vi "TagCreatePixelArrayV1Tags.vi"(5 "Layout":string, 7 "Codes":i64[](array[numeric]), 8 "error in (no error)":errorcluster, 11 "ID":i32) -> (0 "error out":errorcluster, 3 "Pixels":u8[][](array[numeric]))   [LabVIEW 2020, in "g_ar_toolkit.feature_detection.lvlib"]
uses:
  g_ar_toolkit.feature_detection.lvlib
  TagPixelType.ctl
  <vilib>/Utility/error.llb/Error Cluster From Error Code.vi
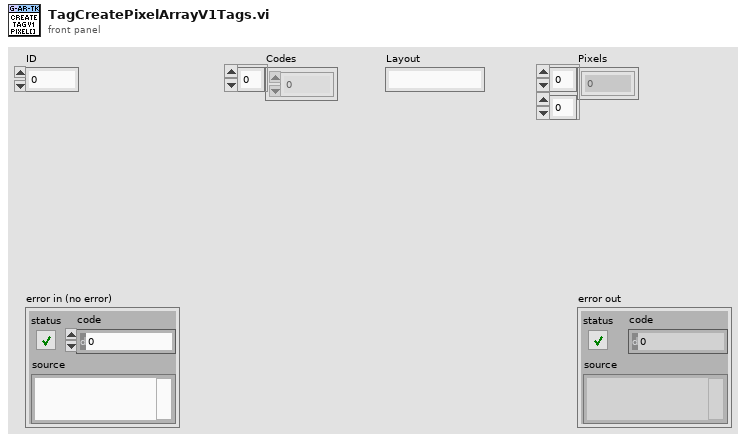
[diagram p1: front panel]
types:
  T1 = typedef "g_ar_toolkit.feature_detection.lvlib/TagPixelType.ctl" = enum8{"Black", "White", "Transparent"}
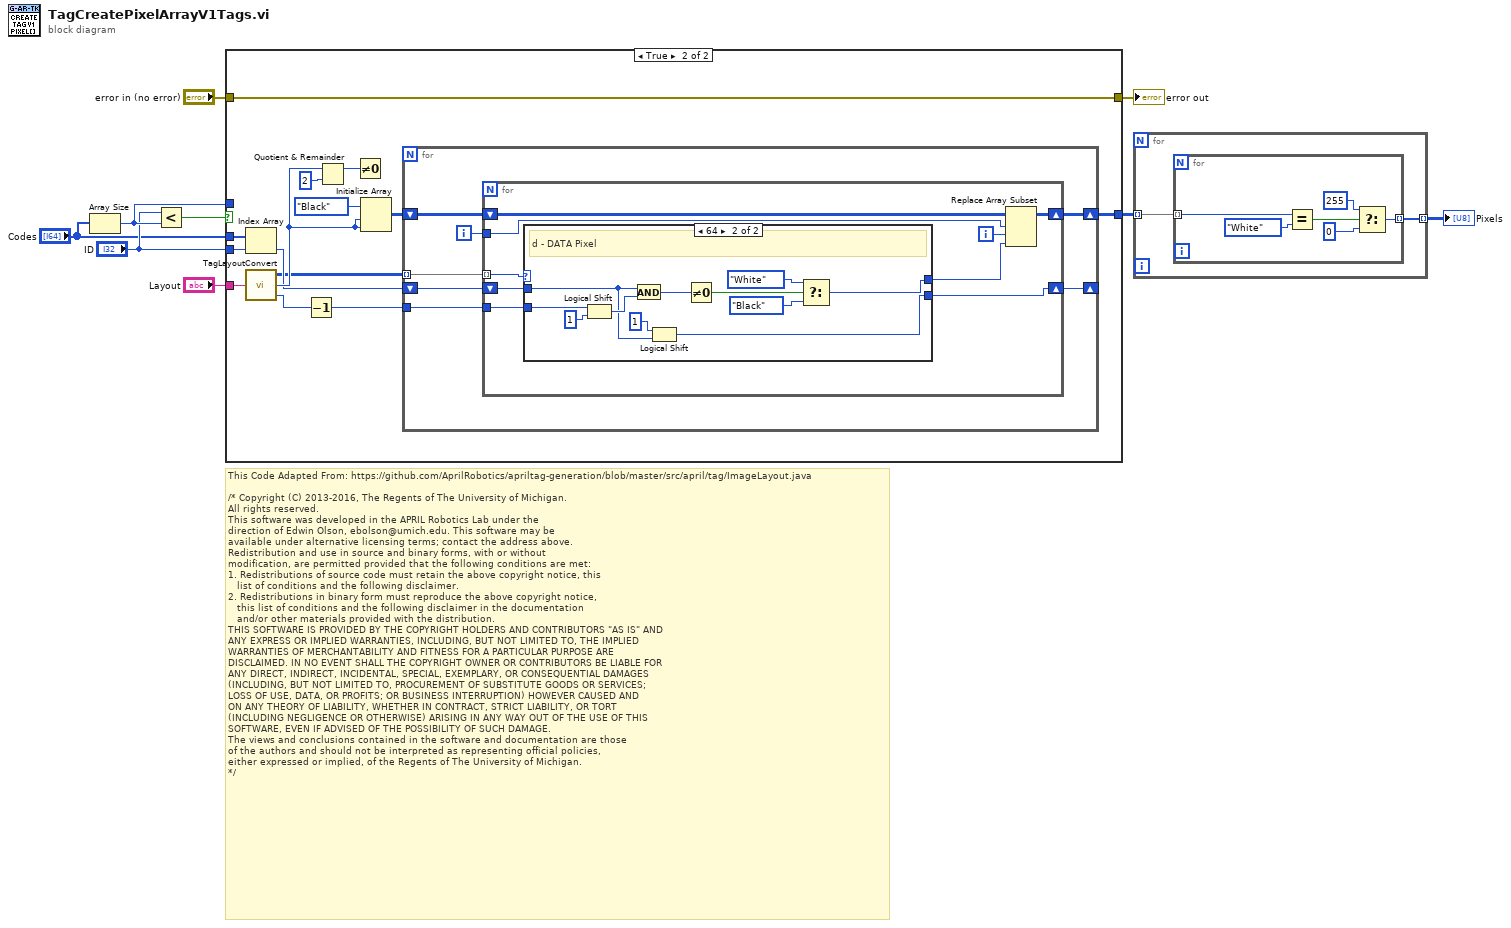
[diagram p0: block diagram]
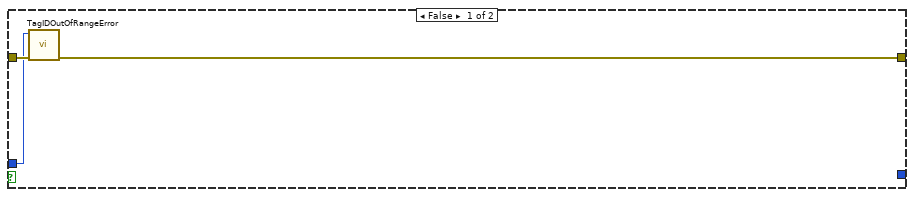
[diagram p2: hidden frame]
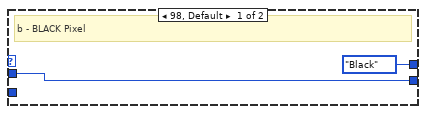
[diagram p3: hidden frame]
diagram:
  # "This Code Adapted From: https://github.com/AprilRobotics/apriltag-generation/blob/master/src/april/tag/ImageLayout.java\n\n/* Copyright (C) 2013-2016, The Regents of The University of Michigan.\nAll rights reserved.\nThis software was developed in the APRIL Robotics Lab under the\ndirection of Edwin Olson, ebolson@umich.edu. This software may be\navailable under alternative licensing terms; contact the address above.\nRedistribution and use in source and binary forms, with or without\nmodification, are permitted provided that the following conditions are met:\n1. Redistributions of source code must retain the above copyright notice, this\n   list of conditions and the following disclaimer.\n2. Redistributions in binary form must reproduce the above copyright notice,\n   this list of conditions and the following disclaimer in the documentation\n   and/or other materials provided with the distribution.\nTHIS SOFTWARE IS PROVIDED BY THE COPYRIGHT HOLDERS AND CONTRIBUTORS \"AS IS\" AND\nANY EXPRESS OR IMPLIED WARRANTIES, INCLUDING, BUT NOT LIMITED TO, THE IMPLIED\nWARRANTIES OF MERCHANTABILITY AND FITNESS FOR A PARTICULAR PURPOSE ARE\nDISCLAIMED. IN NO EVENT SHALL THE COPYRIGHT OWNER OR CONTRIBUTORS BE LIABLE FOR\nANY DIRECT, INDIRECT, INCIDENTAL, SPECIAL, EXEMPLARY, OR CONSEQUENTIAL DAMAGES\n(INCLUDING, BUT NOT LIMITED TO, PROCUREMENT OF SUBSTITUTE GOODS OR SERVICES;\nLOSS OF USE, DATA, OR PROFITS; OR BUSINESS INTERRUPTION) HOWEVER CAUSED AND\nON ANY THEORY OF LIABILITY, WHETHER IN CONTRACT, STRICT LIABILITY, OR TORT\n(INCLUDING NEGLIGENCE OR OTHERWISE) ARISING IN ANY WAY OUT OF THE USE OF THIS\nSOFTWARE, EVEN IF ADVISED OF THE POSSIBILITY OF SUCH DAMAGE.\nThe views and conclusions contained in the software and documentation are those\nof the authors and should not be interpreted as representing official policies,\neither expressed or implied, of the Regents of The University of Michigan.\n*/"
  n1 = Array Size(array="Codes") -> (size(s)=w8:i32)
  n2 = Less?(x="ID", y=w8) -> (x < y?=w5:bool)
  n3 = case shown="True" w5 {
    tunnel: "Codes" -> [_ w26]
    tunnel: "ID" -> [_ w25]
    tunnel: "error in (no error)" -> [w12 w19]
    tunnel: [w11 w19] -> w7
    tunnel: w8 -> [w10 _]
    tunnel: "Layout" -> [_ w21]
    tunnel: [_ w13] -> w2
    frame False {
      n4 = call "TagIDOutOfRangeError.vi"("error in (no error)"=w12, "Tag Family Size"=w10) -> ("error out"=w11:errorcluster)  [unwired: 9 in]
    }
    frame True {
      n5 = Index Array(array=w26, index=w25) -> (element=w18:i64)
      n6 = call "TagLayoutConvert.vi"("Layout"=w21) -> ("Pixel Map"=w17:u8[][], "Size"=w20:i32, "Number Of Bits"=w15:i32)
      n7 = Decrement(x=w15) -> (x-1=w14:i32)
      n8 = Quotient & Remainder(x=w20, y=2) -> (x-y*floor(x/y)=w23:i32)  [unwired: 1 out]
      n9 = Not Equal To 0?(x=w23) -> ()  [unwired: 1 out]
      n10 = Initialize Array(TagPixelType."Black", w20, w20) -> (w16:T1[][])
      n11 = for {
        shift-right: [w28] -> _
        shift-left: w18 -> [w29]
        tunnel: w17 -> [w33] mode=indexing
        shift-right: [w27] -> w13
        shift-left: w16 -> [w32]
        tunnel: w14 -> [w30]
        i -> [w31]
        n12 = for {
          tunnel: w33 -> [w42] mode=indexing
          shift-right: [w40] -> w27
          shift-left: w32 -> [w41]
          tunnel: w31 -> [w38]
          tunnel: w30 -> [w36]
          shift-right: [w34] -> w28
          shift-left: w29 -> [w35]
          i -> [w37]
          n13 = case shown="64" w42 {
            tunnel: [TagPixelType."Black" ("TagPixelType") w49] -> w39
            tunnel: [w43 w53] -> w34
            tunnel: w36 -> [_ w46]
            tunnel: w35 -> [w43 w45]
            frame 98, Default {
              # "b - BLACK Pixel"
            }
            frame 100 {
              # "d - DATA Pixel"
              n14 = Logical Shift(y=w46, x=i64 1) -> (x << y=w55:i64)
              n15 = And(x=w45, y=w55) -> (x .and. y?=w54:i64)
              n16 = Logical Shift(y=i16 1, x=w45) -> (x << y=w53:i64)
              n17 = Not Equal To 0?(x=w54) -> (x != 0?=w50:bool)
              n18 = Select(t=TagPixelType."White" ("TagPixelType"), s=w50, f=TagPixelType."Black") -> (s? t:f=w49:T1)
            }
          }
          n19 = Replace Array Subset(array=w41, new element=w39, index (row)=w38, index (col)=w37) -> (w40:T1[][])
        }
      }
    }
  }
  "error out" <- w7
  n20 = for {
    tunnel: w2 -> [w57] mode=indexing
    tunnel: [w56] -> w1 mode=indexing
    n21 = for {
      tunnel: w57 -> [w63] mode=indexing
      tunnel: [w59] -> w56 mode=indexing
      n22 = Equal?(x=w63, y=TagPixelType."White") -> (x = y?=w61:bool)
      n23 = Select(t=u8 255, s=w61, f=u8 0) -> (s? t:f=w59:u8)
    }
  }
  "Pixels" <- w1
